vi "Final_StolenBreaker.vi"() -> ()   [LabVIEW 2014]
uses:
  <vilib>/DAQmx/create/channels.llb/DAQmx Create Channel (CO-Pulse Generation-Frequency).vi
  <vilib>/DAQmx/configure/timing.llb/DAQmx Timing (Implicit).vi
  <vilib>/DAQmx/write.llb/DAQmx Write (Counter Frequency 1Chan 1Samp).vi
  <vilib>/DAQmx/create/channels.llb/DAQmx Create Channel (DO-Digital Output).vi
  <vilib>/DAQmx/write.llb/DAQmx Write (Digital Bool 1Line 1Point).vi
  <vilib>/express/express arith-compare/Formula/XNode/ExpressFormulaBlockNode.xnode
panel:
  out "Elapsed Time (s)":dbl
  out "Numeric 2":dbl
  in  "Phase Selection":string(combo)
  in  "Time Target (s)":dbl=1e-08
  in  "frequency":dbl=1.0 format="%_6g"
  out "Numeric":dbl
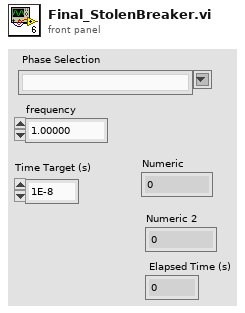
[diagram p1: front panel]
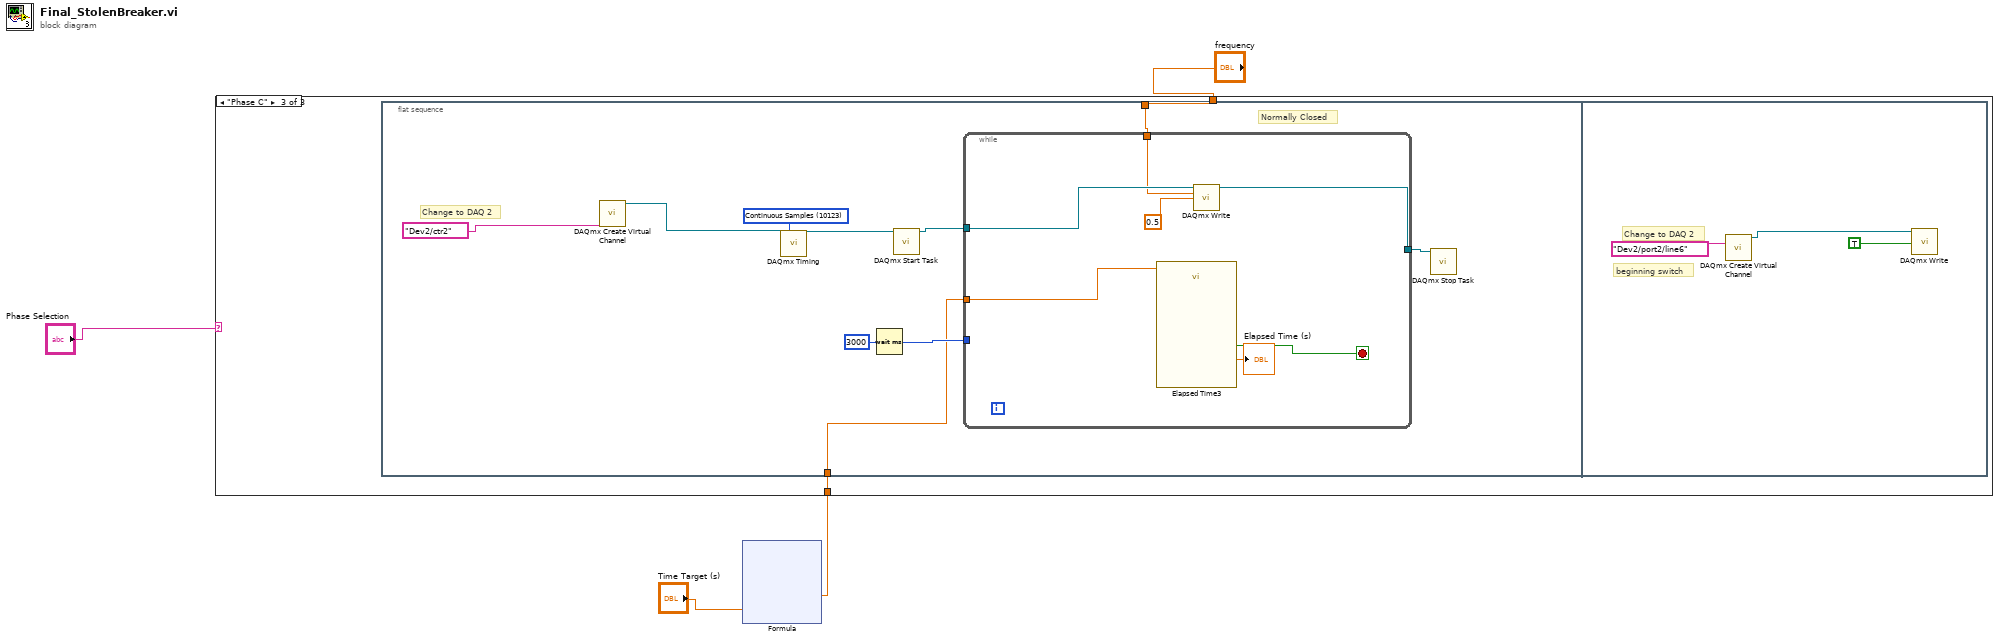
[diagram p0: block diagram]
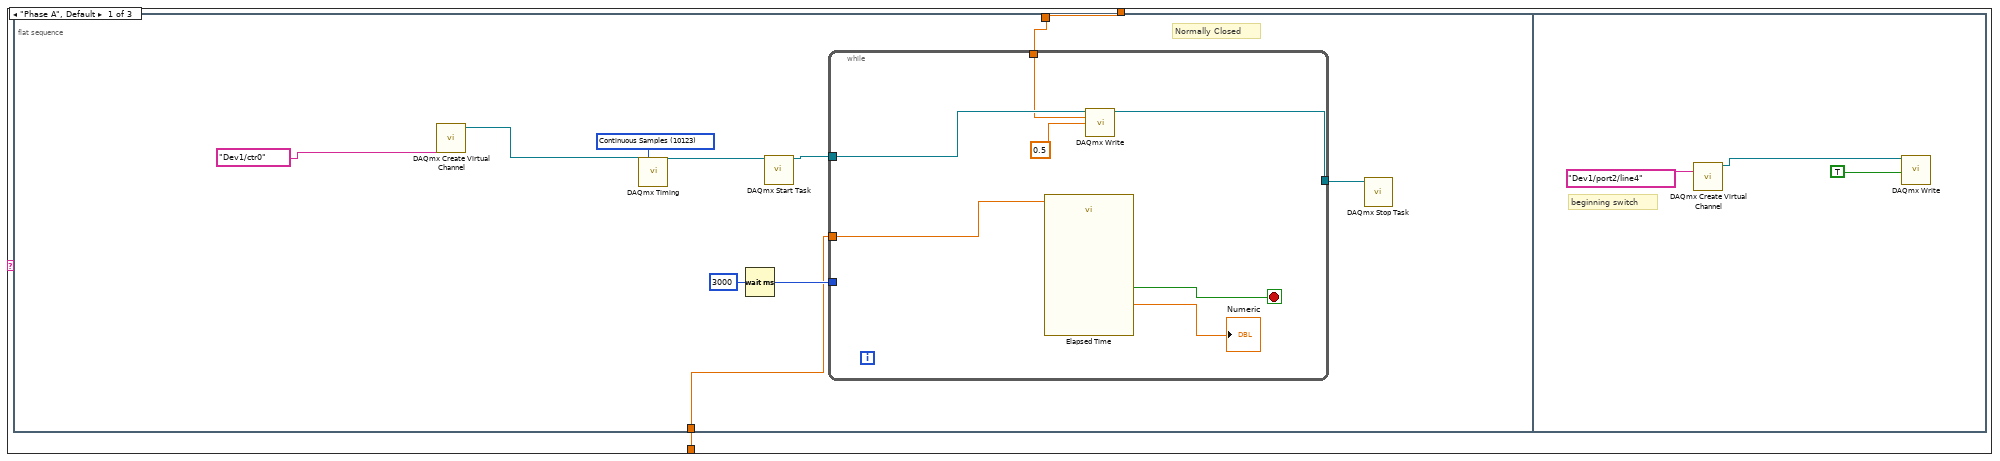
[diagram p2: hidden frame]
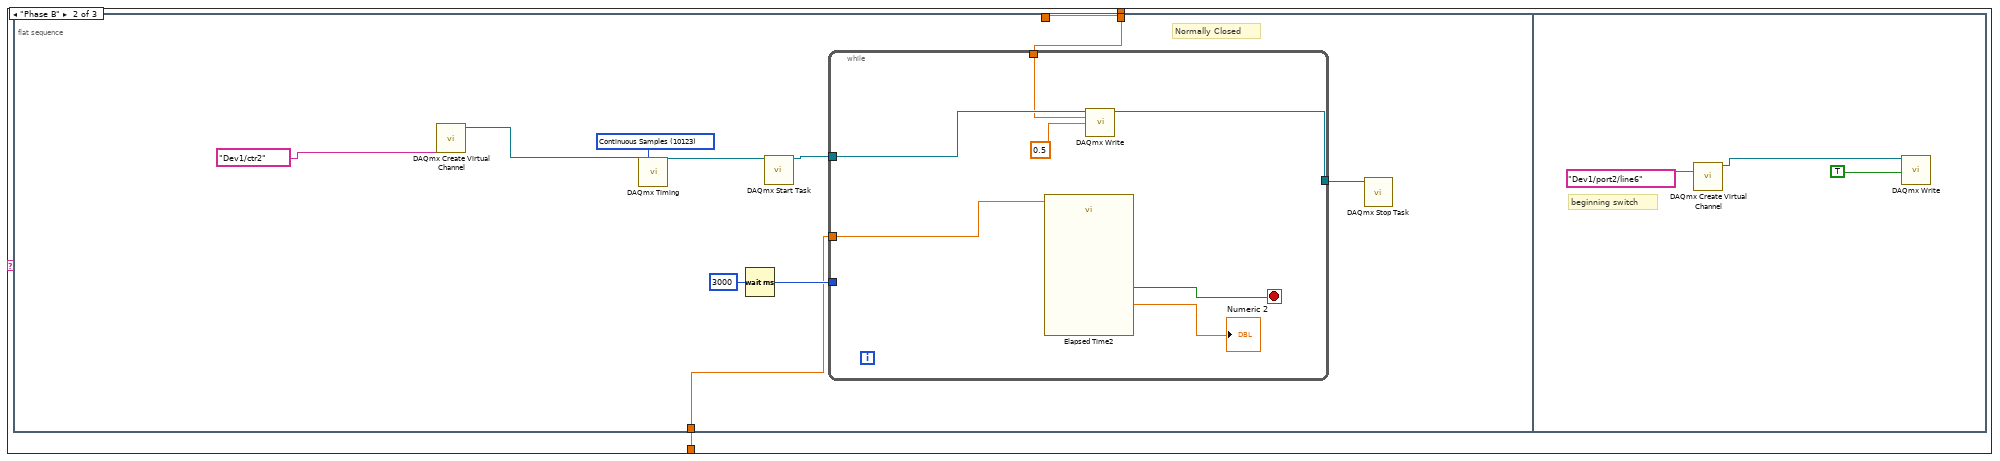
[diagram p3: hidden frame]
diagram:
  n1 = xnode "Formula"("X"="Time Target (s)") -> ("Result"=w2:dbl)  [unwired: 1 in, 1 out]
  n2 = case shown="\"Phase C\"" "Phase Selection" {
    tunnel: w2 -> [w6 w28 w50]
    tunnel: "frequency" -> [w5 w27 w49]
    frame "Phase A", Default {
      n3 = flat-sequence {
        tunnel: w6 -> [w8]
        tunnel: w5 -> [w7]
        frame #0 {
          w16 = 10123 items=["Finite Samples"=10178, "Continuous Samples"=10123, "Hardware Timed Single Point"=12522] ("sample mode")
          # "Normally Closed"
          n4 = call-poly <vilib>:"DAQmx Create Virtual Channel.vi"("counter"=tag "Dev1/ctr0") -> ("task out"=w11:refnum<k21>)  [unwired: 8 in, 6 out]
          n5 = call-poly <vilib>:"DAQmx Timing.vi"("task/channels in"=w11, "sample mode"=w16) -> ("task out"=w12:refnum<k21>)  [unwired: 4 in, 9 out]
          n6 = Wait (ms)(milliseconds to wait=u32 3000) -> (millisecond timer value=w14:u32)
          n7 = call <vilib>:"DAQmx Start Task.vi"("task/channels in"=w12) -> ("task out"=w15:refnum<k21>)  [unwired: 1 in, 13 out]
          n8 = while {
            tunnel: w15 -> [w22]
            tunnel: w14 -> [_]
            tunnel: w8 -> [w19]
            tunnel: [w18] -> w10
            tunnel: w7 -> [w17]
            stop <- w20 stop-if-true
            n9 = call "Elapsed Time"("Time Target (s)"=w19) -> ("Elapsed Time (s)"=→"Numeric":dbl, "Time has Elapsed"=w20:bool)  [unwired: 11 in, 6 out]
            n10 = call-poly <vilib>:"DAQmx Write.vi"("task/channels in"=w22, "frequency"=w17, "duty cycle"=0.5) -> ("task out"=w18:refnum<k21>)  [unwired: 2 in, 10 out]
          }
          n11 = call <vilib>:"DAQmx Stop Task.vi"("task/channels in"=w10) -> ()  [unwired: 13 in, 2 out]
        }
        frame #1 {
          # "beginning switch"
          n12 = call-poly <vilib>:"DAQmx Create Virtual Channel.vi"("lines"=tag "Dev1/port2/line4") -> ("task out"=w26:refnum<k21>)  [unwired: 13 in, 1 out]
          n13 = call-poly <vilib>:"DAQmx Write.vi"("task/channels in"=w26, "data"=TRUE) -> ()  [unwired: 11 in, 3 out]
        }
      }
    }
    frame "Phase B" {
      n14 = flat-sequence {
        tunnel: w28 -> [w30]
        tunnel: w27 -> [_]
        tunnel: w27 -> [w29]
        frame #0 {
          w38 = 10123 items=["Finite Samples"=10178, "Continuous Samples"=10123, "Hardware Timed Single Point"=12522] ("sample mode")
          # "Normally Closed"
          n15 = call-poly <vilib>:"DAQmx Create Virtual Channel.vi"("counter"=tag "Dev1/ctr2") -> ("task out"=w33:refnum<k21>)  [unwired: 8 in, 6 out]
          n16 = call-poly <vilib>:"DAQmx Timing.vi"("task/channels in"=w33, "sample mode"=w38) -> ("task out"=w34:refnum<k21>)  [unwired: 4 in, 9 out]
          n17 = Wait (ms)(milliseconds to wait=u32 3000) -> (millisecond timer value=w36:u32)
          n18 = call <vilib>:"DAQmx Start Task.vi"("task/channels in"=w34) -> ("task out"=w37:refnum<k21>)  [unwired: 1 in, 13 out]
          n19 = while {
            tunnel: w37 -> [w44]
            tunnel: w36 -> [_]
            tunnel: w30 -> [w41]
            tunnel: [w40] -> w32
            tunnel: w29 -> [w39]
            stop <- w42 stop-if-true
            n20 = call "Elapsed Time2"("Time Target (s)"=w41) -> ("Elapsed Time (s)"=→"Numeric 2":dbl, "Time has Elapsed"=w42:bool)  [unwired: 11 in, 6 out]
            n21 = call-poly <vilib>:"DAQmx Write.vi"("task/channels in"=w44, "frequency"=w39, "duty cycle"=0.5) -> ("task out"=w40:refnum<k21>)  [unwired: 2 in, 10 out]
          }
          n22 = call <vilib>:"DAQmx Stop Task.vi"("task/channels in"=w32) -> ()  [unwired: 13 in, 2 out]
        }
        frame #1 {
          # "beginning switch"
          n23 = call-poly <vilib>:"DAQmx Create Virtual Channel.vi"("lines"=tag "Dev1/port2/line6") -> ("task out"=w48:refnum<k21>)  [unwired: 13 in, 1 out]
          n24 = call-poly <vilib>:"DAQmx Write.vi"("task/channels in"=w48, "data"=TRUE) -> ()  [unwired: 11 in, 3 out]
        }
      }
    }
    frame "Phase C" {
      n25 = flat-sequence {
        tunnel: w50 -> [w52]
        tunnel: w49 -> [w51]
        frame #0 {
          w60 = 10123 items=["Finite Samples"=10178, "Continuous Samples"=10123, "Hardware Timed Single Point"=12522] ("sample mode")
          # "Change to DAQ 2"
          # "Normally Closed"
          n26 = call-poly <vilib>:"DAQmx Create Virtual Channel.vi"("counter"=tag "Dev2/ctr2") -> ("task out"=w55:refnum<k21>)  [unwired: 8 in, 6 out]
          n27 = call-poly <vilib>:"DAQmx Timing.vi"("task/channels in"=w55, "sample mode"=w60) -> ("task out"=w56:refnum<k21>)  [unwired: 4 in, 9 out]
          n28 = Wait (ms)(milliseconds to wait=u32 3000) -> (millisecond timer value=w58:u32)
          n29 = call <vilib>:"DAQmx Start Task.vi"("task/channels in"=w56) -> ("task out"=w59:refnum<k21>)  [unwired: 1 in, 13 out]
          n30 = while {
            tunnel: w59 -> [w66]
            tunnel: w58 -> [_]
            tunnel: w52 -> [w64]
            tunnel: [w63] -> w54
            tunnel: w51 -> [w62]
            stop <- w65 stop-if-true
            n31 = call "Elapsed Time3"("Time Target (s)"=w64) -> ("Elapsed Time (s)"=→"Elapsed Time (s)":dbl, "Time has Elapsed"=w65:bool)  [unwired: 11 in, 6 out]
            n32 = call-poly <vilib>:"DAQmx Write.vi"("task/channels in"=w66, "frequency"=w62, "duty cycle"=0.5) -> ("task out"=w63:refnum<k21>)  [unwired: 2 in, 10 out]
          }
          n33 = call <vilib>:"DAQmx Stop Task.vi"("task/channels in"=w54) -> ()  [unwired: 13 in, 2 out]
        }
        frame #1 {
          # "Change to DAQ 2"
          # "beginning switch"
          n34 = call-poly <vilib>:"DAQmx Create Virtual Channel.vi"("lines"=tag "Dev2/port2/line6") -> ("task out"=w70:refnum<k21>)  [unwired: 13 in, 1 out]
          n35 = call-poly <vilib>:"DAQmx Write.vi"("task/channels in"=w70, "data"=TRUE) -> ()  [unwired: 11 in, 3 out]
        }
      }
    }
  }
